vi "Begin.vi"(8 "error in":errorcluster) -> (0 "error out":errorcluster)   [LabVIEW 2017]
doc: "Called before other user functions, this VI is expected to open initial I/O refnums, load in file data, and do all program initialization. Notice that the <B>error out</B> terminal is simply used for data flow. Wiring it to other structures or subVIs ensures that this VI runs first."
uses:
  <vilib>/Rock Robotics/WPI/DriverStation/WPI_DriverStationRobotMode2.ctl
  TypeDef/CLUSTER_Arm_Device_IDs.ctl
  TypeDef/CLUSTER_Talon_Setup.ctl
  _SHARE ALL/RoboRio Share All/SRX Share All/TypeDefs SRX/Cluster_SRX_OPEN Data.ctl
  _SHARE ALL/RoboRio Share All/SRX Share All/TypeDefs SRX/Cluster_SRX_Current Config.ctl
  _SHARE ALL/RoboRio Share All/SRX Share All/TypeDefs SRX/Cluster_SRX_Sensor Config.ctl
  System Drivers/Phoenix-LabVIEW/Motor Controller/Controls/CTRE_Phoenix_MotorControl_FeedbackDevice.ctl
  _SHARE ALL/RoboRio Share All/SRX Share All/TypeDefs SRX/Cluster_SRX_Config Hard Limits.ctl
  System Drivers/Phoenix-LabVIEW/Motor Controller/Controls/CTRE_Phoenix_MotorControl_LimitSwitchNormal.ctl
  _SHARE ALL/RoboRio Share All/SRX Share All/TypeDefs SRX/Cluster_SRX_Motion Magic Config Data.ctl
  _SHARE ALL/RoboRio Share All/SRX Share All/TypeDefs SRX/Cluster_SRX_PIDF.ctl
  _SHARE ALL/RoboRio Share All/SRX Share All/TypeDefs SRX/Cluster_SRX_Config Soft Limits.ctl
  _SHARE ALL/RoboRio Share All/SRX Share All/TypeDefs SRX/Cluster_SRX_Config Voltage Output.ctl
  System Drivers/Phoenix-LabVIEW/Motor Controller/Controls/CTRE_Phoenix_MotorControl_NeutralMode.ctl
  _SHARE ALL/RoboRio Share All/SRX Share All/TypeDefs SRX/Cluster_SRX_Forward and Reverse.ctl
  TypeDef/CLUSTER_Claw_Setup.ctl
  TypeDef/CLUSTER_PWM Motor Setup.ctl
  TypeDef/CLUSTER_Solonoid_Setup.ctl
  <vilib>/Rock Robotics/WPI/Solenoid/WPI_SolenoidChannel.ctl
  <vilib>/Rock Robotics/SystemInterfaces/DIO/FPGA_DIOChannel.ctl
  TypeDef/CLUSTER_Drive_Setup.ctl
  Robot Global Data.vi
  _SHARE ALL/Global Share All/Global_STOP.vi
  Globals/Global_Device_IDs.vi
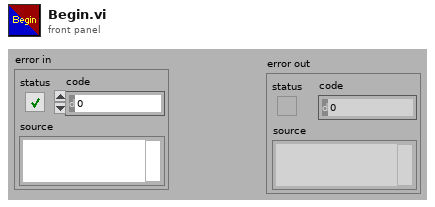
[diagram p1: front panel]
types:
  T1 = typedef "WPI_DriverStationRobotMode2.ctl" = enum16{"Autonomous Disabled", "Autonomous Enabled", "Teleop Disabled", "Teleop Enabled", "Disconnected", "Finish", "Test Disabled", "Test Enabled", "Emergency Stopped"}
  T2 = typedef "CTRE_Phoenix_MotorControl_LimitSwitchNormal.ctl" = enum16{"Normally Open", "Normally Closed", "Disabled"}
  T3 = typedef "Cluster_SRX_Config Hard Limits.ctl" = cluster{"Fwd Enable":bool, "Rev Enable":bool, "Fwd NO-NC":T2, "Rev NO-NC":T2}
  T4 = typedef "Cluster_SRX_Forward and Reverse.ctl" = cluster{"Forward":dbl, "Reverse":dbl}
  T5 = typedef "CTRE_Phoenix_MotorControl_NeutralMode.ctl" = enum8{"EEPROMSetting", "Override to Coast", "Override to Brake"}
  T6 = typedef "Cluster_SRX_Config Voltage Output.ctl" = cluster{"Invert?":bool, "Neutral Mode":T5, "Deadband (-1to1)":dbl, "Ramp Time Off to Full (S)":dbl, "Peak  (-1to1)":T4, "Nominal  (-1to1)":T4}
  T7 = typedef "Cluster_SRX_Config Soft Limits.ctl" = cluster{"Max":i32, "Min":i32, "Max Enable":bool, "Min Enable":bool}
  T8 = typedef "Cluster_SRX_PIDF.ctl" = cluster{"P":dbl, "I":dbl, "D":dbl, "F":dbl, "I Zone":dbl}
  T9 = typedef "Cluster_SRX_Sensor Config.ctl" = cluster{"Feedback Device":T10, "PhaseSensor":bool}
  T10 = typedef "CTRE_Phoenix_MotorControl_FeedbackDevice.ctl" = i8
  T11 = typedef "Cluster_SRX_OPEN Data.ctl" = cluster{"SRX ID":u8, "Invert Output":bool}
  T12 = typedef "CLUSTER_Talon_Setup.ctl" = cluster{"Open Data":T11, "Current Config Data":T13, "Sensor Config":T9, "Hard Limits":T3, "Motion Magic Config Data":T14, "PIDF":T8, "Maximum Integral Accumulator Value":dbl, "AllowableClosedLoop":i32, "Limits":T7, "Output Config":T6}
  T13 = typedef "Cluster_SRX_Current Config.ctl" = cluster{"Enable Current Limit?":bool, "Peak Current (Amps)":i32, "Peak Current Maximum Duration (ms)":i32, "Continuous Current Limit (Amps)":i32}
  T14 = typedef "Cluster_SRX_Motion Magic Config Data.ctl" = cluster{"Cruise Velocity":i32, "Acceleration":i32}
  T15 = typedef "CLUSTER_Arm_Device_IDs.ctl" = cluster{"Master":T12, "Slave":T12}
  T16 = typedef "CLUSTER_Drive_Setup.ctl" = cluster{"Left Master":T12, "Right Master":T12, "Left Slave":T12, "Right Slave":T12}
  T17 = typedef "FPGA_DIOChannel.ctl" = enum8{"DIO 0", "DIO 1", "DIO 2", "DIO 3", "DIO 4", "DIO 5", "DIO 6", "DIO 7", "DIO 8", "DIO 9", "DIO MXP 0", "DIO MXP 1", "DIO MXP 2", "DIO MXP 3", "DIO MXP 4", "DIO MXP 5", "DIO MXP 6", "DIO MXP 7", "DIO MXP 8", "DIO MXP 9", "DIO MXP 10", "DIO MXP 11", "DIO MXP 12", "DIO MXP 13", "DIO MXP 14", "DIO MXP 15", "SPI Port CS1", "SPI Port CS2", "SPI Port CS3", "SPI Port MISO", "SPI Port MOSI", "Invalid"}
  T18 = typedef "WPI_SolenoidChannel.ctl" = enum8{"Solenoid 0", "Solenoid 1", "Solenoid 2", "Solenoid 3", "Solenoid 4", "Solenoid 5", "Solenoid 6", "Solenoid 7", "Invalid"}
  T19 = typedef "CLUSTER_Claw_Setup.ctl" = cluster{"Left Motor Setup":T20, "Right Motor Setup":T20, "Left Motor PDP":i32, "Right Motor PDP":i32, "Solonoid Setup":T21, "Limit Switch DIO":T17}
  T20 = typedef "CLUSTER_PWM Motor Setup.ctl" = cluster{"Motor ID":u8, "Invert Motor":bool}
  T21 = typedef "CLUSTER_Solonoid_Setup.ctl" = cluster{"Pneumatics Control Module (0)":u8, "Forward Solenoid Channel":T18, "Reverse Solenoid Channel":T18}
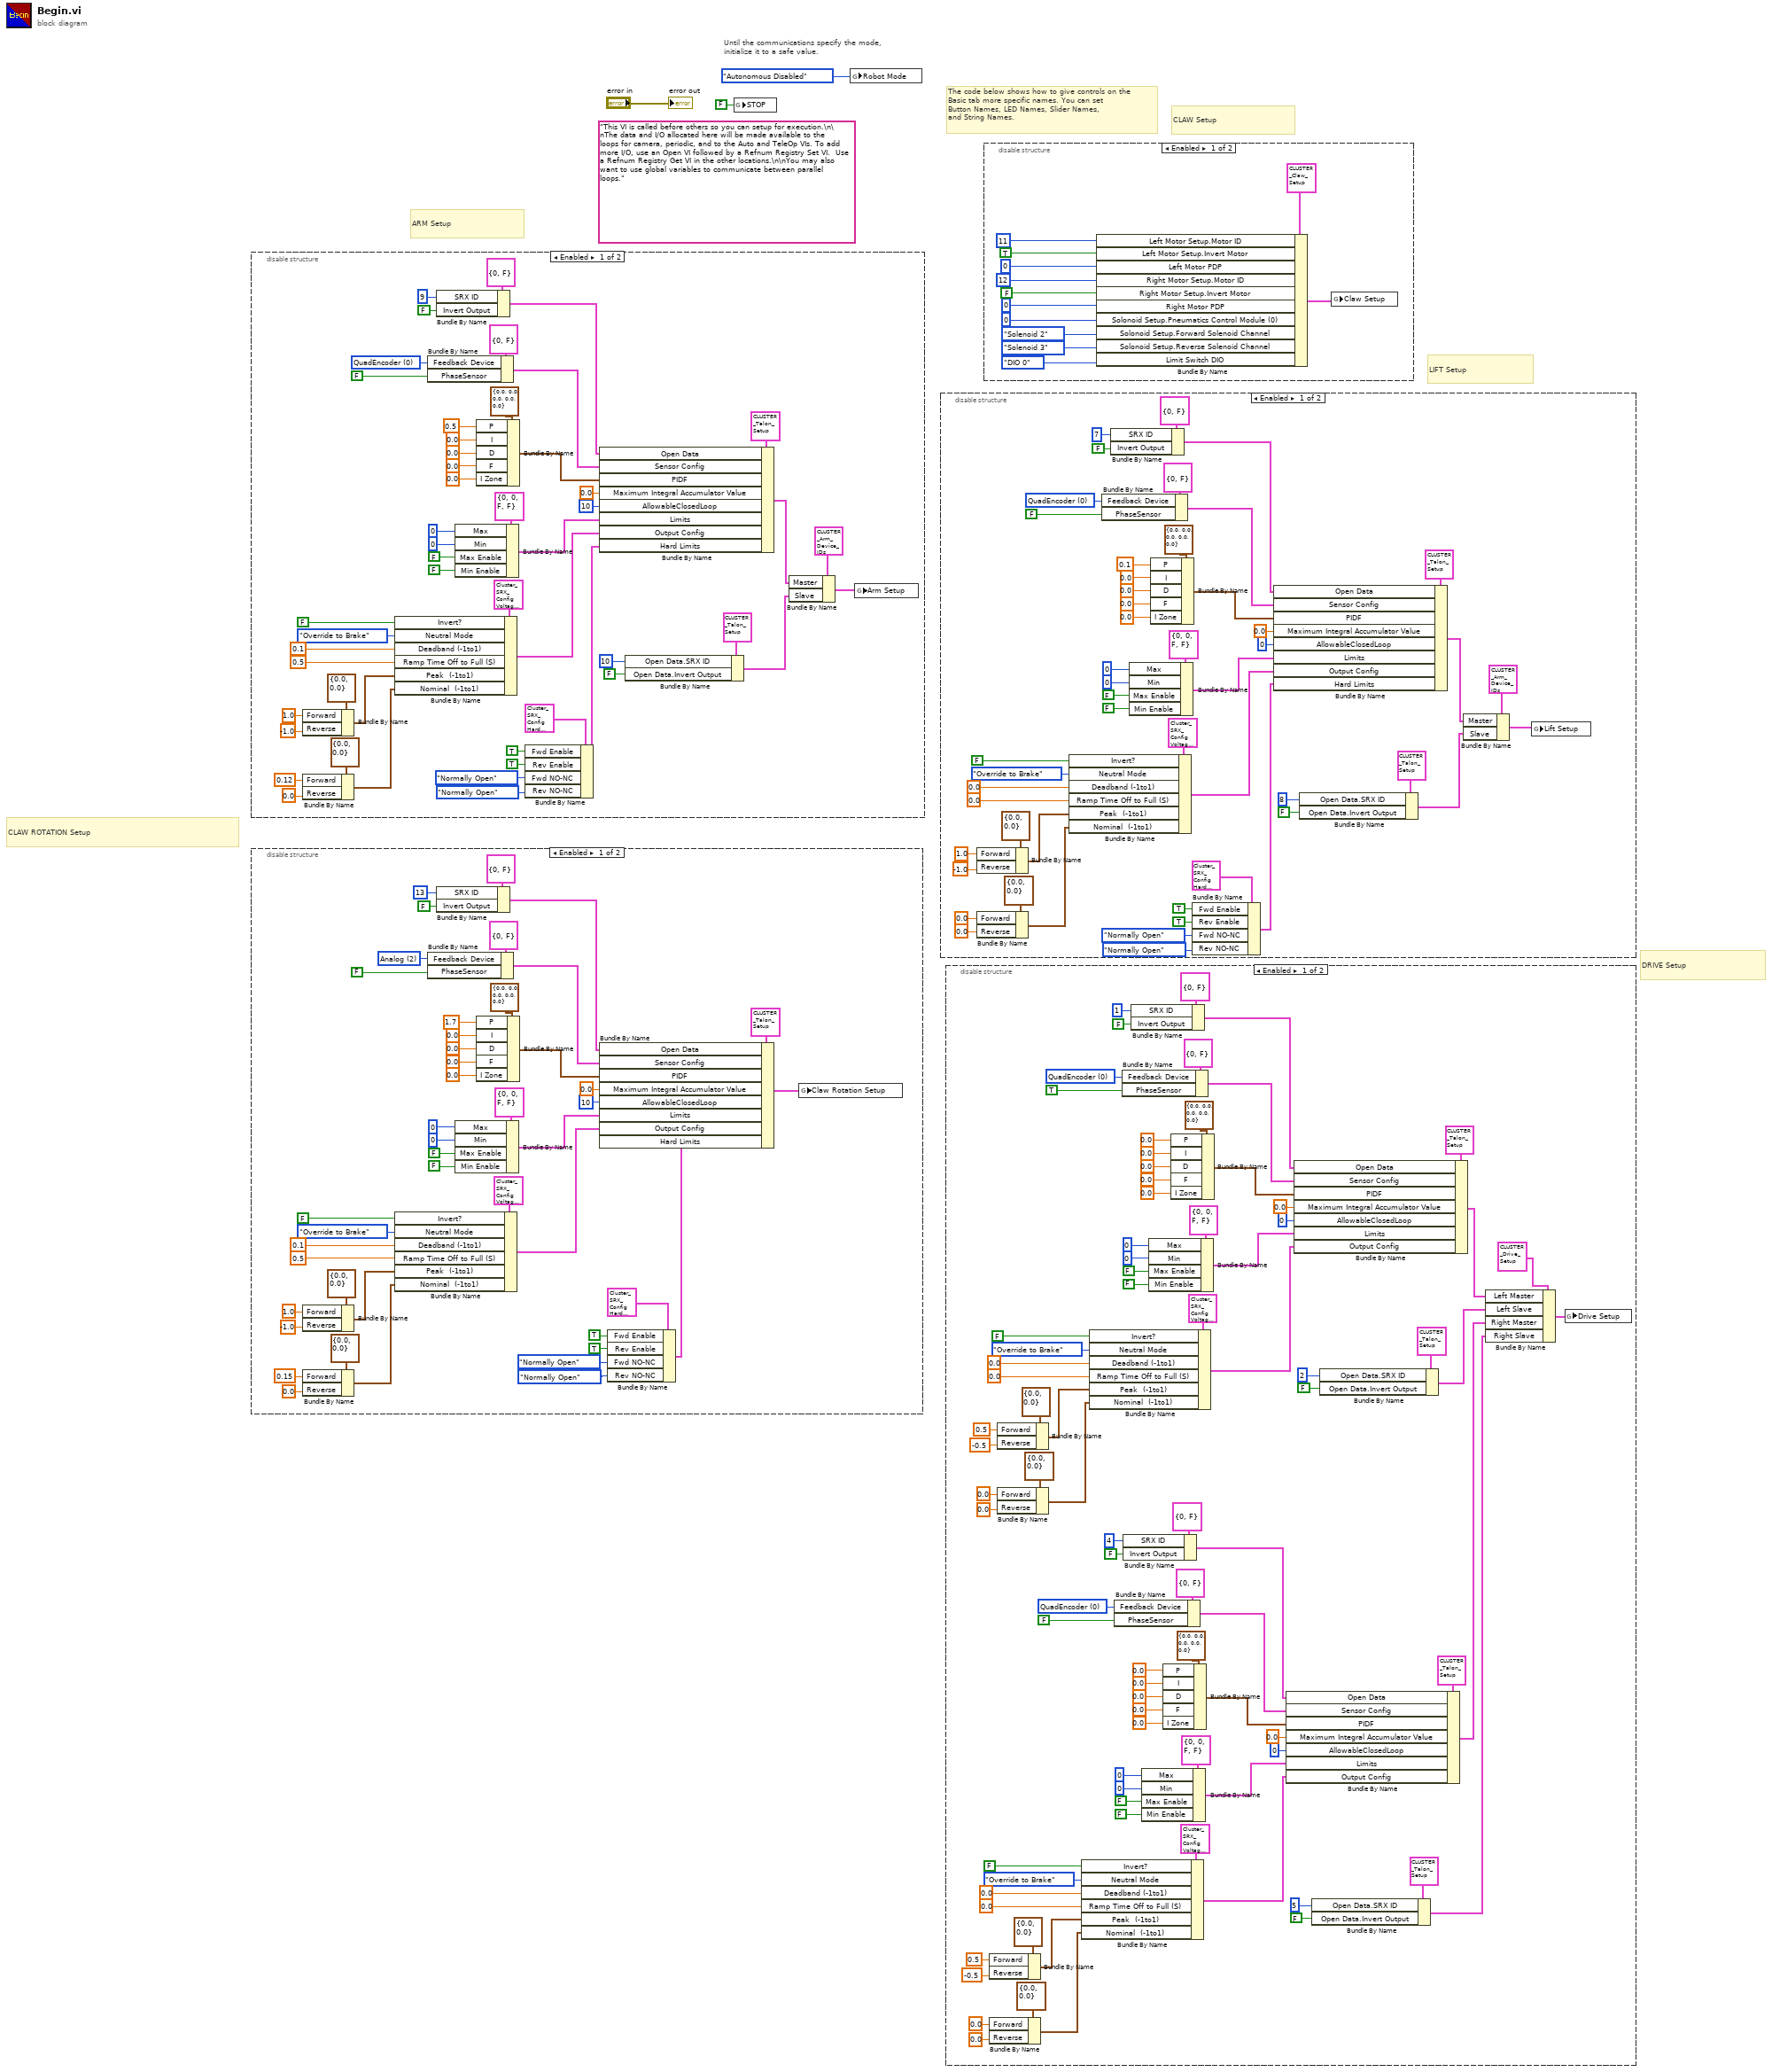
[diagram p0: block diagram]
diagram:
  (unwired) "This VI is called before others so you can setup for execution.\n\nThe data and I/O allocated here will be made available to the loops for camera, periodic, and to the Auto and TeleOp VIs. To add more I/O, use an Open VI followed by a Refnum Registry Set VI.  Use a Refnum Registry Get VI in the other locations.\n\nYou may also want to use global variables to communicate between parallel loops."
  # "DRIVE Setup"
  # "CLAW ROTATION Setup"
  # "LIFT Setup"
  # "CLAW Setup"
  # "ARM Setup"
  # "The code below shows how to give controls on the\nBasic tab more specific names. You can set\nButton Names, LED Names, Slider Names,\nand String Names."
  # "Until the communications specify the mode,\ninitialize it to a safe value."
  n1 = disable-structure shown="Enabled" {
    frame Enabled {
      w34 = T10 0 items=["None"=-1, "QuadEncoder"=0, "Analog"=2, "Tachometer"=4, "Pulse Width Encoded Position"=8, "Sensor Sum (S0 + S1)"=9, "Sensor Difference (D0 - D1)"=10, "Remote Source 0"=11, "Remote Source 1"=12, "Software Emulated"=15] ("Feedback Device")
      n2 = Bundle By Name(cluster=T4 {"Forward"=0.0, "Reverse"=0.0} ("Peak  (-1to1)"), "Forward"=1.0, "Reverse"=-1.0) -> (w18:T4)
      n3 = Bundle By Name(cluster=T4 {"Forward"=0.0, "Reverse"=0.0} ("Nominal  (-1to1)"), "Forward"=0.12, "Reverse"=0.0) -> (w16:T4)
      n4 = Bundle By Name(cluster=T6 {"Invert?"=FALSE, "Neutral Mode"=enum."Override to Coast", "Deadband (-1to1)"=0.0, "Ramp Time Off to Full (S)"=0.0, "Peak  (-1to1)"={"Forward"=1.0, "Reverse"=-1.0}, "Nominal  (-1to1)"={"Forward"=0.0, "Reverse"=0.0}} ("Output Config"), "Invert?"=FALSE, "Neutral Mode"=CTRE_Phoenix_MotorControl_NeutralMode."Override to Brake", "Deadband (-1to1)"=0.1, "Ramp Time Off to Full (S)"=0.5, "Peak  (-1to1)"=w18, "Nominal  (-1to1)"=w16) -> (w37:T6)
      n5 = Bundle By Name(cluster=T9 {"Feedback Device"=0, "PhaseSensor"=FALSE} ("Sensor Config"), "Feedback Device"=w34, "PhaseSensor"=FALSE) -> (w45:T9)
      n6 = Bundle By Name(cluster=T11 {"SRX ID"=0, "Invert Output"=FALSE} ("Open Data"), "SRX ID"=u8 9, "Invert Output"=FALSE) -> (w47:T11)
      n7 = Bundle By Name(cluster=T7 {"Max"=0, "Min"=0, "Max Enable"=FALSE, "Min Enable"=FALSE} ("Limits"), "Max"=0, "Min"=0, "Max Enable"=FALSE, "Min Enable"=FALSE) -> (w39:T7)
      n8 = Bundle By Name(cluster=T8 {"P"=0.0, "I"=0.0, "D"=0.0, "F"=0.0, "I Zone"=0.0} ("PIDF"), "P"=0.5, "I"=0.0, "D"=0.0, "F"=0.0, "I Zone"=0.0) -> (w43:T8)
      n9 = Bundle By Name(cluster=T3 {"Fwd Enable"=FALSE, "Rev Enable"=FALSE, "Fwd NO-NC"=enum."Normally Open", "Rev NO-NC"=enum."Normally Open"} ("Hard Limits"), "Fwd Enable"=TRUE, "Rev Enable"=TRUE, "Fwd NO-NC"=CTRE_Phoenix_MotorControl_LimitSwitchNormal."Normally Open", "Rev NO-NC"=CTRE_Phoenix_MotorControl_LimitSwitchNormal."Normally Open") -> (w4:T3)
      n10 = Bundle By Name(cluster=T12 {"Open Data"={"SRX ID"=0, "Invert Output"=FALSE}, "Current Config Data"={"Enable Current Limit?"=FALSE, "Peak Current (Amps)"=0, "Peak Current Maximum Duration (ms)"=0, "Continuous Current Limit (Amps)"=0}, "Sensor Config"={"Feedback Device"=0, "PhaseSensor"=FALSE}, "Hard Limits"={"Fwd Enable"=FALSE, "Rev Enable"=FALSE, "Fwd NO-NC"=enum."Normally Open", "Rev NO-NC"=enum."Normally Open"}, "Motion Magic Config Data"={"Cruise Velocity"=0, "Acceleration"=0}, "PIDF"={"P"=0.0, "I"=0.0, "D"=0.0, "F"=0.0, "I Zone"=0.0}, "Maximum Integral Accumulator Value"=0.0, "AllowableClosedLoop"=0, "Limits"={"Max"=0, "Min"=0, "Max Enable"=FALSE, "Min Enable"=FALSE}, "Output Config"={"Invert?"=FALSE, "Neutral Mode"=enum."Override to Coast", "Deadband (-1to1)"=0.0, "Ramp Time Off to Full (S)"=0.0, "Peak  (-1to1)"={"Forward"=1.0, "Reverse"=-1.0}, "Nominal  (-1to1)"={"Forward"=0.0, "Reverse"=0.0}}} ("Master"), "Open Data"=w47, "Sensor Config"=w45, "PIDF"=w43, "Maximum Integral Accumulator Value"=0.0, "AllowableClosedLoop"=10, "Limits"=w39, "Output Config"=w37, "Hard Limits"=w4) -> (w51:T12)
      n11 = Bundle By Name(cluster=T12 {"Open Data"={"SRX ID"=0, "Invert Output"=FALSE}, "Current Config Data"={"Enable Current Limit?"=FALSE, "Peak Current (Amps)"=0, "Peak Current Maximum Duration (ms)"=0, "Continuous Current Limit (Amps)"=0}, "Sensor Config"={"Feedback Device"=0, "PhaseSensor"=FALSE}, "Hard Limits"={"Fwd Enable"=FALSE, "Rev Enable"=FALSE, "Fwd NO-NC"=enum."Normally Open", "Rev NO-NC"=enum."Normally Open"}, "Motion Magic Config Data"={"Cruise Velocity"=0, "Acceleration"=0}, "PIDF"={"P"=0.0, "I"=0.0, "D"=0.0, "F"=0.0, "I Zone"=0.0}, "Maximum Integral Accumulator Value"=0.0, "AllowableClosedLoop"=0, "Limits"={"Max"=0, "Min"=0, "Max Enable"=FALSE, "Min Enable"=FALSE}, "Output Config"={"Invert?"=FALSE, "Neutral Mode"=enum."Override to Coast", "Deadband (-1to1)"=0.0, "Ramp Time Off to Full (S)"=0.0, "Peak  (-1to1)"={"Forward"=1.0, "Reverse"=-1.0}, "Nominal  (-1to1)"={"Forward"=0.0, "Reverse"=0.0}}} ("Master"), "Open Data.SRX ID"=u8 10, "Open Data.Invert Output"=FALSE) -> (w50:T12)
      n12 = Bundle By Name(cluster=T15 {"Master"={"Open Data"={"SRX ID"=0, "Invert Output"=FALSE}, "Current Config Data"={"Enable Current Limit?"=FALSE, "Peak Current (Amps)"=0, "Peak Current Maximum Duration (ms)"=2, "Continuous Current Limit (Amps)"=0}, "Sensor Config"={"Feedback Device"=0, "PhaseSensor"=FALSE}, "Hard Limits"={"Fwd Enable"=FALSE, "Rev Enable"=FALSE, "Fwd NO-NC"=enum."Normally Open", "Rev NO-NC"=enum."Normally Open"}, "Motion Magic Config Data"={"Cruise Velocity"=0, "Acceleration"=0}, "PIDF"={"P"=0.0, "I"=0.0, "D"=0.0, "F"=0.0, "I Zone"=0.0}, "Maximum Integral Accumulator Value"=0.0, "AllowableClosedLoop"=0, "Limits"={"Max"=0, "Min"=0, "Max Enable"=FALSE, "Min Enable"=FALSE}, "Output Config"={"Invert?"=FALSE, "Neutral Mode"=enum."Override to Coast", "Deadband (-1to1)"=0.0, "Ramp Time Off to Full (S)"=0.0, "Peak  (-1to1)"={"Forward"=1.0, "Reverse"=-1.0}, "Nominal  (-1to1)"={"Forward"=0.0, "Reverse"=0.0}}}, "Slave"={"Open Data"={"SRX ID"=0, "Invert Output"=FALSE}, "Current Config Data"={"Enable Current Limit?"=FALSE, "Peak Current (Amps)"=0, "Peak Current Maximum Duration (ms)"=-1, "Continuous Current Limit (Amps)"=0}, "Sensor Config"={"Feedback Device"=0, "PhaseSensor"=FALSE}, "Hard Limits"={"Fwd Enable"=FALSE, "Rev Enable"=FALSE, "Fwd NO-NC"=enum."Normally Open", "Rev NO-NC"=enum."Normally Open"}, "Motion Magic Config Data"={"Cruise Velocity"=0, "Acceleration"=0}, "PIDF"={"P"=0.0, "I"=0.0, "D"=0.0, "F"=0.0, "I Zone"=0.0}, "Maximum Integral Accumulator Value"=0.0, "AllowableClosedLoop"=0, "Limits"={"Max"=0, "Min"=0, "Max Enable"=FALSE, "Min Enable"=FALSE}, "Output Config"={"Invert?"=FALSE, "Neutral Mode"=enum."Override to Coast", "Deadband (-1to1)"=0.0, "Ramp Time Off to Full (S)"=0.0, "Peak  (-1to1)"={"Forward"=1.0, "Reverse"=-1.0}, "Nominal  (-1to1)"={"Forward"=0.0, "Reverse"=0.0}}}} ("Arm Setup"), "Master"=w51, "Slave"=w50) -> (w53:T15)
      n13 = global write "Global_Device_IDs.vi" "Arm Setup"(w53) -> ()
    }
    frame Disabled {
    }
  }
  n14 = disable-structure shown="Enabled" {
    frame Enabled {
      w84 = T10 2 items=["None"=-1, "QuadEncoder"=0, "Analog"=2, "Tachometer"=4, "Pulse Width Encoded Position"=8, "Sensor Sum (S0 + S1)"=9, "Sensor Difference (D0 - D1)"=10, "Remote Source 0"=11, "Remote Source 1"=12, "Software Emulated"=15] ("Feedback Device")
      n15 = Bundle By Name(cluster=T4 {"Forward"=0.0, "Reverse"=0.0} ("Peak  (-1to1)"), "Forward"=1.0, "Reverse"=-1.0) -> (w68:T4)
      n16 = Bundle By Name(cluster=T4 {"Forward"=0.0, "Reverse"=0.0} ("Nominal  (-1to1)"), "Forward"=0.15, "Reverse"=0.0) -> (w66:T4)
      n17 = Bundle By Name(cluster=T6 {"Invert?"=FALSE, "Neutral Mode"=enum."Override to Coast", "Deadband (-1to1)"=0.0, "Ramp Time Off to Full (S)"=0.0, "Peak  (-1to1)"={"Forward"=1.0, "Reverse"=-1.0}, "Nominal  (-1to1)"={"Forward"=0.0, "Reverse"=0.0}} ("Output Config"), "Invert?"=FALSE, "Neutral Mode"=CTRE_Phoenix_MotorControl_NeutralMode."Override to Brake", "Deadband (-1to1)"=0.1, "Ramp Time Off to Full (S)"=0.5, "Peak  (-1to1)"=w68, "Nominal  (-1to1)"=w66) -> (w87:T6)
      n18 = Bundle By Name(cluster=T9 {"Feedback Device"=0, "PhaseSensor"=FALSE} ("Sensor Config"), "Feedback Device"=w84, "PhaseSensor"=FALSE) -> (w95:T9)
      n19 = Bundle By Name(cluster=T11 {"SRX ID"=0, "Invert Output"=FALSE} ("Open Data"), "SRX ID"=u8 13, "Invert Output"=FALSE) -> (w97:T11)
      n20 = Bundle By Name(cluster=T7 {"Max"=0, "Min"=0, "Max Enable"=FALSE, "Min Enable"=FALSE} ("Limits"), "Max"=0, "Min"=0, "Max Enable"=FALSE, "Min Enable"=FALSE) -> (w89:T7)
      n21 = Bundle By Name(cluster=T8 {"P"=0.0, "I"=0.0, "D"=0.0, "F"=0.0, "I Zone"=0.0} ("PIDF"), "P"=1.7, "I"=0.0, "D"=0.0, "F"=0.0, "I Zone"=0.0) -> (w93:T8)
      n22 = Bundle By Name(cluster=T3 {"Fwd Enable"=FALSE, "Rev Enable"=FALSE, "Fwd NO-NC"=enum."Normally Open", "Rev NO-NC"=enum."Normally Open"} ("Hard Limits"), "Fwd Enable"=TRUE, "Rev Enable"=TRUE, "Fwd NO-NC"=CTRE_Phoenix_MotorControl_LimitSwitchNormal."Normally Open", "Rev NO-NC"=CTRE_Phoenix_MotorControl_LimitSwitchNormal."Normally Open") -> (w56:T3)
      n23 = Bundle By Name(cluster=T12 {"Open Data"={"SRX ID"=0, "Invert Output"=FALSE}, "Current Config Data"={"Enable Current Limit?"=FALSE, "Peak Current (Amps)"=0, "Peak Current Maximum Duration (ms)"=0, "Continuous Current Limit (Amps)"=0}, "Sensor Config"={"Feedback Device"=0, "PhaseSensor"=FALSE}, "Hard Limits"={"Fwd Enable"=FALSE, "Rev Enable"=FALSE, "Fwd NO-NC"=enum."Normally Open", "Rev NO-NC"=enum."Normally Open"}, "Motion Magic Config Data"={"Cruise Velocity"=0, "Acceleration"=0}, "PIDF"={"P"=0.0, "I"=0.0, "D"=0.0, "F"=0.0, "I Zone"=0.0}, "Maximum Integral Accumulator Value"=0.0, "AllowableClosedLoop"=0, "Limits"={"Max"=0, "Min"=0, "Max Enable"=FALSE, "Min Enable"=FALSE}, "Output Config"={"Invert?"=FALSE, "Neutral Mode"=enum."Override to Coast", "Deadband (-1to1)"=0.0, "Ramp Time Off to Full (S)"=0.0, "Peak  (-1to1)"={"Forward"=1.0, "Reverse"=-1.0}, "Nominal  (-1to1)"={"Forward"=0.0, "Reverse"=0.0}}} ("Master"), "Open Data"=w97, "Sensor Config"=w95, "PIDF"=w93, "Maximum Integral Accumulator Value"=0.0, "AllowableClosedLoop"=10, "Limits"=w89, "Output Config"=w87, "Hard Limits"=w56) -> (w61:T12)
      n24 = global write "Global_Device_IDs.vi" "Claw Rotation Setup"(w61) -> ()
    }
    frame Disabled {
    }
  }
  n25 = global write "Global_STOP.vi" "STOP"(FALSE ("STOP")) -> ()
  n26 = global write "Robot Global Data.vi" "Robot Mode"(WPI_DriverStationRobotMode2."Autonomous Disabled" ("Robot Mode")) -> ()
  n27 = disable-structure shown="Enabled" {
    frame Enabled {
      w130 = T10 0 items=["None"=-1, "QuadEncoder"=0, "Analog"=2, "Tachometer"=4, "Pulse Width Encoded Position"=8, "Sensor Sum (S0 + S1)"=9, "Sensor Difference (D0 - D1)"=10, "Remote Source 0"=11, "Remote Source 1"=12, "Software Emulated"=15] ("Feedback Device")
      n28 = Bundle By Name(cluster=T4 {"Forward"=0.0, "Reverse"=0.0} ("Peak  (-1to1)"), "Forward"=1.0, "Reverse"=-1.0) -> (w114:T4)
      n29 = Bundle By Name(cluster=T4 {"Forward"=0.0, "Reverse"=0.0} ("Nominal  (-1to1)"), "Forward"=0.0, "Reverse"=0.0) -> (w112:T4)
      n30 = Bundle By Name(cluster=T6 {"Invert?"=FALSE, "Neutral Mode"=enum."Override to Coast", "Deadband (-1to1)"=0.0, "Ramp Time Off to Full (S)"=0.0, "Peak  (-1to1)"={"Forward"=1.0, "Reverse"=-1.0}, "Nominal  (-1to1)"={"Forward"=0.0, "Reverse"=0.0}} ("Output Config"), "Invert?"=FALSE, "Neutral Mode"=CTRE_Phoenix_MotorControl_NeutralMode."Override to Brake", "Deadband (-1to1)"=0.0, "Ramp Time Off to Full (S)"=0.0, "Peak  (-1to1)"=w114, "Nominal  (-1to1)"=w112) -> (w133:T6)
      n31 = Bundle By Name(cluster=T9 {"Feedback Device"=0, "PhaseSensor"=FALSE} ("Sensor Config"), "Feedback Device"=w130, "PhaseSensor"=FALSE) -> (w141:T9)
      n32 = Bundle By Name(cluster=T11 {"SRX ID"=0, "Invert Output"=FALSE} ("Open Data"), "SRX ID"=u8 7, "Invert Output"=FALSE) -> (w143:T11)
      n33 = Bundle By Name(cluster=T7 {"Max"=0, "Min"=0, "Max Enable"=FALSE, "Min Enable"=FALSE} ("Limits"), "Max"=0, "Min"=0, "Max Enable"=FALSE, "Min Enable"=FALSE) -> (w135:T7)
      n34 = Bundle By Name(cluster=T8 {"P"=0.0, "I"=0.0, "D"=0.0, "F"=0.0, "I Zone"=0.0} ("PIDF"), "P"=0.1, "I"=0.0, "D"=0.0, "F"=0.0, "I Zone"=0.0) -> (w139:T8)
      n35 = Bundle By Name(cluster=T3 {"Fwd Enable"=FALSE, "Rev Enable"=FALSE, "Fwd NO-NC"=enum."Normally Open", "Rev NO-NC"=enum."Normally Open"} ("Hard Limits"), "Fwd Enable"=TRUE, "Rev Enable"=TRUE, "Fwd NO-NC"=CTRE_Phoenix_MotorControl_LimitSwitchNormal."Normally Open", "Rev NO-NC"=CTRE_Phoenix_MotorControl_LimitSwitchNormal."Normally Open") -> (w105:T3)
      n36 = Bundle By Name(cluster=T12 {"Open Data"={"SRX ID"=0, "Invert Output"=FALSE}, "Current Config Data"={"Enable Current Limit?"=FALSE, "Peak Current (Amps)"=0, "Peak Current Maximum Duration (ms)"=0, "Continuous Current Limit (Amps)"=0}, "Sensor Config"={"Feedback Device"=0, "PhaseSensor"=FALSE}, "Hard Limits"={"Fwd Enable"=FALSE, "Rev Enable"=FALSE, "Fwd NO-NC"=enum."Normally Open", "Rev NO-NC"=enum."Normally Open"}, "Motion Magic Config Data"={"Cruise Velocity"=0, "Acceleration"=0}, "PIDF"={"P"=0.0, "I"=0.0, "D"=0.0, "F"=0.0, "I Zone"=0.0}, "Maximum Integral Accumulator Value"=0.0, "AllowableClosedLoop"=0, "Limits"={"Max"=0, "Min"=0, "Max Enable"=FALSE, "Min Enable"=FALSE}, "Output Config"={"Invert?"=FALSE, "Neutral Mode"=enum."Override to Coast", "Deadband (-1to1)"=0.0, "Ramp Time Off to Full (S)"=0.0, "Peak  (-1to1)"={"Forward"=1.0, "Reverse"=-1.0}, "Nominal  (-1to1)"={"Forward"=0.0, "Reverse"=0.0}}} ("Master"), "Open Data"=w143, "Sensor Config"=w141, "PIDF"=w139, "Maximum Integral Accumulator Value"=0.0, "AllowableClosedLoop"=0, "Limits"=w135, "Output Config"=w133, "Hard Limits"=w105) -> (w147:T12)
      n37 = Bundle By Name(cluster=T12 {"Open Data"={"SRX ID"=0, "Invert Output"=FALSE}, "Current Config Data"={"Enable Current Limit?"=FALSE, "Peak Current (Amps)"=0, "Peak Current Maximum Duration (ms)"=0, "Continuous Current Limit (Amps)"=0}, "Sensor Config"={"Feedback Device"=0, "PhaseSensor"=FALSE}, "Hard Limits"={"Fwd Enable"=FALSE, "Rev Enable"=FALSE, "Fwd NO-NC"=enum."Normally Open", "Rev NO-NC"=enum."Normally Open"}, "Motion Magic Config Data"={"Cruise Velocity"=0, "Acceleration"=0}, "PIDF"={"P"=0.0, "I"=0.0, "D"=0.0, "F"=0.0, "I Zone"=0.0}, "Maximum Integral Accumulator Value"=0.0, "AllowableClosedLoop"=0, "Limits"={"Max"=0, "Min"=0, "Max Enable"=FALSE, "Min Enable"=FALSE}, "Output Config"={"Invert?"=FALSE, "Neutral Mode"=enum."Override to Coast", "Deadband (-1to1)"=0.0, "Ramp Time Off to Full (S)"=0.0, "Peak  (-1to1)"={"Forward"=1.0, "Reverse"=-1.0}, "Nominal  (-1to1)"={"Forward"=0.0, "Reverse"=0.0}}} ("Master"), "Open Data.SRX ID"=u8 8, "Open Data.Invert Output"=FALSE) -> (w146:T12)
      n38 = Bundle By Name(cluster=T15 {"Master"={"Open Data"={"SRX ID"=0, "Invert Output"=FALSE}, "Current Config Data"={"Enable Current Limit?"=FALSE, "Peak Current (Amps)"=0, "Peak Current Maximum Duration (ms)"=2, "Continuous Current Limit (Amps)"=0}, "Sensor Config"={"Feedback Device"=0, "PhaseSensor"=FALSE}, "Hard Limits"={"Fwd Enable"=FALSE, "Rev Enable"=FALSE, "Fwd NO-NC"=enum."Normally Open", "Rev NO-NC"=enum."Normally Open"}, "Motion Magic Config Data"={"Cruise Velocity"=0, "Acceleration"=0}, "PIDF"={"P"=0.0, "I"=0.0, "D"=0.0, "F"=0.0, "I Zone"=0.0}, "Maximum Integral Accumulator Value"=0.0, "AllowableClosedLoop"=0, "Limits"={"Max"=0, "Min"=0, "Max Enable"=FALSE, "Min Enable"=FALSE}, "Output Config"={"Invert?"=FALSE, "Neutral Mode"=enum."Override to Coast", "Deadband (-1to1)"=0.0, "Ramp Time Off to Full (S)"=0.0, "Peak  (-1to1)"={"Forward"=1.0, "Reverse"=-1.0}, "Nominal  (-1to1)"={"Forward"=0.0, "Reverse"=0.0}}}, "Slave"={"Open Data"={"SRX ID"=0, "Invert Output"=FALSE}, "Current Config Data"={"Enable Current Limit?"=FALSE, "Peak Current (Amps)"=0, "Peak Current Maximum Duration (ms)"=-1, "Continuous Current Limit (Amps)"=0}, "Sensor Config"={"Feedback Device"=0, "PhaseSensor"=FALSE}, "Hard Limits"={"Fwd Enable"=FALSE, "Rev Enable"=FALSE, "Fwd NO-NC"=enum."Normally Open", "Rev NO-NC"=enum."Normally Open"}, "Motion Magic Config Data"={"Cruise Velocity"=0, "Acceleration"=0}, "PIDF"={"P"=0.0, "I"=0.0, "D"=0.0, "F"=0.0, "I Zone"=0.0}, "Maximum Integral Accumulator Value"=0.0, "AllowableClosedLoop"=0, "Limits"={"Max"=0, "Min"=0, "Max Enable"=FALSE, "Min Enable"=FALSE}, "Output Config"={"Invert?"=FALSE, "Neutral Mode"=enum."Override to Coast", "Deadband (-1to1)"=0.0, "Ramp Time Off to Full (S)"=0.0, "Peak  (-1to1)"={"Forward"=1.0, "Reverse"=-1.0}, "Nominal  (-1to1)"={"Forward"=0.0, "Reverse"=0.0}}}} ("Arm Setup"), "Master"=w147, "Slave"=w146) -> (w149:T15)
      n39 = global write "Global_Device_IDs.vi" "Lift Setup"(w149) -> ()
    }
    frame Disabled {
    }
  }
  n40 = disable-structure shown="Enabled" {
    frame Enabled {
      w170 = T10 0 items=["None"=-1, "QuadEncoder"=0, "Analog"=2, "Tachometer"=4, "Pulse Width Encoded Position"=8, "Sensor Sum (S0 + S1)"=9, "Sensor Difference (D0 - D1)"=10, "Remote Source 0"=11, "Remote Source 1"=12, "Software Emulated"=15] ("Feedback Device")
      w220 = T10 0 items=["None"=-1, "QuadEncoder"=0, "Analog"=2, "Tachometer"=4, "Pulse Width Encoded Position"=8, "Sensor Sum (S0 + S1)"=9, "Sensor Difference (D0 - D1)"=10, "Remote Source 0"=11, "Remote Source 1"=12, "Software Emulated"=15] ("Feedback Device")
      n41 = Bundle By Name(cluster=T4 {"Forward"=0.0, "Reverse"=0.0} ("Peak  (-1to1)"), "Forward"=0.5, "Reverse"=-0.5) -> (w186:T4)
      n42 = Bundle By Name(cluster=T4 {"Forward"=0.0, "Reverse"=0.0} ("Nominal  (-1to1)"), "Forward"=0.0, "Reverse"=0.0) -> (w188:T4)
      n43 = Bundle By Name(cluster=T4 {"Forward"=0.0, "Reverse"=0.0} ("Peak  (-1to1)"), "Forward"=0.5, "Reverse"=-0.5) -> (w204:T4)
      n44 = Bundle By Name(cluster=T4 {"Forward"=0.0, "Reverse"=0.0} ("Nominal  (-1to1)"), "Forward"=0.0, "Reverse"=0.0) -> (w202:T4)
      n45 = Bundle By Name(cluster=T6 {"Invert?"=FALSE, "Neutral Mode"=enum."Override to Coast", "Deadband (-1to1)"=0.0, "Ramp Time Off to Full (S)"=0.0, "Peak  (-1to1)"={"Forward"=1.0, "Reverse"=-1.0}, "Nominal  (-1to1)"={"Forward"=0.0, "Reverse"=0.0}} ("Output Config"), "Invert?"=FALSE, "Neutral Mode"=CTRE_Phoenix_MotorControl_NeutralMode."Override to Brake", "Deadband (-1to1)"=0.0, "Ramp Time Off to Full (S)"=0.0, "Peak  (-1to1)"=w186, "Nominal  (-1to1)"=w188) -> (w167:T6)
      n46 = Bundle By Name(cluster=T6 {"Invert?"=FALSE, "Neutral Mode"=enum."Override to Coast", "Deadband (-1to1)"=0.0, "Ramp Time Off to Full (S)"=0.0, "Peak  (-1to1)"={"Forward"=1.0, "Reverse"=-1.0}, "Nominal  (-1to1)"={"Forward"=0.0, "Reverse"=0.0}} ("Output Config"), "Invert?"=FALSE, "Neutral Mode"=CTRE_Phoenix_MotorControl_NeutralMode."Override to Brake", "Deadband (-1to1)"=0.0, "Ramp Time Off to Full (S)"=0.0, "Peak  (-1to1)"=w204, "Nominal  (-1to1)"=w202) -> (w223:T6)
      n47 = Bundle By Name(cluster=T9 {"Feedback Device"=0, "PhaseSensor"=FALSE} ("Sensor Config"), "Feedback Device"=w170, "PhaseSensor"=FALSE) -> (w159:T9)
      n48 = Bundle By Name(cluster=T9 {"Feedback Device"=0, "PhaseSensor"=FALSE} ("Sensor Config"), "Feedback Device"=w220, "PhaseSensor"=TRUE) -> (w231:T9)
      n49 = Bundle By Name(cluster=T11 {"SRX ID"=0, "Invert Output"=FALSE} ("Open Data"), "SRX ID"=u8 4, "Invert Output"=FALSE) -> (w157:T11)
      n50 = Bundle By Name(cluster=T11 {"SRX ID"=0, "Invert Output"=FALSE} ("Open Data"), "SRX ID"=u8 1, "Invert Output"=FALSE) -> (w233:T11)
      n51 = Bundle By Name(cluster=T7 {"Max"=0, "Min"=0, "Max Enable"=FALSE, "Min Enable"=FALSE} ("Limits"), "Max"=0, "Min"=0, "Max Enable"=FALSE, "Min Enable"=FALSE) -> (w165:T7)
      n52 = Bundle By Name(cluster=T7 {"Max"=0, "Min"=0, "Max Enable"=FALSE, "Min Enable"=FALSE} ("Limits"), "Max"=0, "Min"=0, "Max Enable"=FALSE, "Min Enable"=FALSE) -> (w225:T7)
      n53 = Bundle By Name(cluster=T8 {"P"=0.0, "I"=0.0, "D"=0.0, "F"=0.0, "I Zone"=0.0} ("PIDF"), "P"=0.0, "I"=0.0, "D"=0.0, "F"=0.0, "I Zone"=0.0) -> (w161:T8)
      n54 = Bundle By Name(cluster=T8 {"P"=0.0, "I"=0.0, "D"=0.0, "F"=0.0, "I Zone"=0.0} ("PIDF"), "P"=0.0, "I"=0.0, "D"=0.0, "F"=0.0, "I Zone"=0.0) -> (w229:T8)
      n55 = Bundle By Name(cluster=T12 {"Open Data"={"SRX ID"=0, "Invert Output"=FALSE}, "Current Config Data"={"Enable Current Limit?"=FALSE, "Peak Current (Amps)"=0, "Peak Current Maximum Duration (ms)"=0, "Continuous Current Limit (Amps)"=0}, "Sensor Config"={"Feedback Device"=0, "PhaseSensor"=FALSE}, "Hard Limits"={"Fwd Enable"=FALSE, "Rev Enable"=FALSE, "Fwd NO-NC"=enum."Normally Open", "Rev NO-NC"=enum."Normally Open"}, "Motion Magic Config Data"={"Cruise Velocity"=0, "Acceleration"=0}, "PIDF"={"P"=0.0, "I"=0.0, "D"=0.0, "F"=0.0, "I Zone"=0.0}, "Maximum Integral Accumulator Value"=0.0, "AllowableClosedLoop"=0, "Limits"={"Max"=0, "Min"=0, "Max Enable"=FALSE, "Min Enable"=FALSE}, "Output Config"={"Invert?"=FALSE, "Neutral Mode"=enum."Override to Coast", "Deadband (-1to1)"=0.0, "Ramp Time Off to Full (S)"=0.0, "Peak  (-1to1)"={"Forward"=1.0, "Reverse"=-1.0}, "Nominal  (-1to1)"={"Forward"=0.0, "Reverse"=0.0}}} ("Master"), "Open Data"=w157, "Sensor Config"=w159, "PIDF"=w161, "Maximum Integral Accumulator Value"=0.0, "AllowableClosedLoop"=0, "Limits"=w165, "Output Config"=w167) -> (w153:T12)
      n56 = Bundle By Name(cluster=T12 {"Open Data"={"SRX ID"=0, "Invert Output"=FALSE}, "Current Config Data"={"Enable Current Limit?"=FALSE, "Peak Current (Amps)"=0, "Peak Current Maximum Duration (ms)"=0, "Continuous Current Limit (Amps)"=0}, "Sensor Config"={"Feedback Device"=0, "PhaseSensor"=FALSE}, "Hard Limits"={"Fwd Enable"=FALSE, "Rev Enable"=FALSE, "Fwd NO-NC"=enum."Normally Open", "Rev NO-NC"=enum."Normally Open"}, "Motion Magic Config Data"={"Cruise Velocity"=0, "Acceleration"=0}, "PIDF"={"P"=0.0, "I"=0.0, "D"=0.0, "F"=0.0, "I Zone"=0.0}, "Maximum Integral Accumulator Value"=0.0, "AllowableClosedLoop"=0, "Limits"={"Max"=0, "Min"=0, "Max Enable"=FALSE, "Min Enable"=FALSE}, "Output Config"={"Invert?"=FALSE, "Neutral Mode"=enum."Override to Coast", "Deadband (-1to1)"=0.0, "Ramp Time Off to Full (S)"=0.0, "Peak  (-1to1)"={"Forward"=1.0, "Reverse"=-1.0}, "Nominal  (-1to1)"={"Forward"=0.0, "Reverse"=0.0}}} ("Master"), "Open Data"=w233, "Sensor Config"=w231, "PIDF"=w229, "Maximum Integral Accumulator Value"=0.0, "AllowableClosedLoop"=0, "Limits"=w225, "Output Config"=w223) -> (w237:T12)
      n57 = Bundle By Name(cluster=T12 {"Open Data"={"SRX ID"=0, "Invert Output"=FALSE}, "Current Config Data"={"Enable Current Limit?"=FALSE, "Peak Current (Amps)"=0, "Peak Current Maximum Duration (ms)"=0, "Continuous Current Limit (Amps)"=0}, "Sensor Config"={"Feedback Device"=0, "PhaseSensor"=FALSE}, "Hard Limits"={"Fwd Enable"=FALSE, "Rev Enable"=FALSE, "Fwd NO-NC"=enum."Normally Open", "Rev NO-NC"=enum."Normally Open"}, "Motion Magic Config Data"={"Cruise Velocity"=0, "Acceleration"=0}, "PIDF"={"P"=0.0, "I"=0.0, "D"=0.0, "F"=0.0, "I Zone"=0.0}, "Maximum Integral Accumulator Value"=0.0, "AllowableClosedLoop"=0, "Limits"={"Max"=0, "Min"=0, "Max Enable"=FALSE, "Min Enable"=FALSE}, "Output Config"={"Invert?"=FALSE, "Neutral Mode"=enum."Override to Coast", "Deadband (-1to1)"=0.0, "Ramp Time Off to Full (S)"=0.0, "Peak  (-1to1)"={"Forward"=1.0, "Reverse"=-1.0}, "Nominal  (-1to1)"={"Forward"=0.0, "Reverse"=0.0}}} ("Master"), "Open Data.SRX ID"=u8 5, "Open Data.Invert Output"=FALSE) -> (w152:T12)
      n58 = Bundle By Name(cluster=T12 {"Open Data"={"SRX ID"=0, "Invert Output"=FALSE}, "Current Config Data"={"Enable Current Limit?"=FALSE, "Peak Current (Amps)"=0, "Peak Current Maximum Duration (ms)"=0, "Continuous Current Limit (Amps)"=0}, "Sensor Config"={"Feedback Device"=0, "PhaseSensor"=FALSE}, "Hard Limits"={"Fwd Enable"=FALSE, "Rev Enable"=FALSE, "Fwd NO-NC"=enum."Normally Open", "Rev NO-NC"=enum."Normally Open"}, "Motion Magic Config Data"={"Cruise Velocity"=0, "Acceleration"=0}, "PIDF"={"P"=0.0, "I"=0.0, "D"=0.0, "F"=0.0, "I Zone"=0.0}, "Maximum Integral Accumulator Value"=0.0, "AllowableClosedLoop"=0, "Limits"={"Max"=0, "Min"=0, "Max Enable"=FALSE, "Min Enable"=FALSE}, "Output Config"={"Invert?"=FALSE, "Neutral Mode"=enum."Override to Coast", "Deadband (-1to1)"=0.0, "Ramp Time Off to Full (S)"=0.0, "Peak  (-1to1)"={"Forward"=1.0, "Reverse"=-1.0}, "Nominal  (-1to1)"={"Forward"=0.0, "Reverse"=0.0}}} ("Master"), "Open Data.SRX ID"=u8 2, "Open Data.Invert Output"=FALSE) -> (w236:T12)
      n59 = Bundle By Name(cluster=T16 {"Left Master"={"Open Data"={"SRX ID"=0, "Invert Output"=FALSE}, "Current Config Data"={"Enable Current Limit?"=FALSE, "Peak Current (Amps)"=0, "Peak Current Maximum Duration (ms)"=0, "Continuous Current Limit (Amps)"=0}, "Sensor Config"={"Feedback Device"=1, "PhaseSensor"=FALSE}, "Hard Limits"={"Fwd Enable"=FALSE, "Rev Enable"=FALSE, "Fwd NO-NC"=enum."Normally Open", "Rev NO-NC"=enum."Normally Open"}, "Motion Magic Config Data"={"Cruise Velocity"=0, "Acceleration"=0}, "PIDF"={"P"=0.0, "I"=0.0, "D"=0.0, "F"=0.0, "I Zone"=0.0}, "Maximum Integral Accumulator Value"=0.0, "AllowableClosedLoop"=0, "Limits"={"Max"=0, "Min"=0, "Max Enable"=FALSE, "Min Enable"=FALSE}, "Output Config"={"Invert?"=FALSE, "Neutral Mode"=enum."EEPROMSetting", "Deadband (-1to1)"=0.0, "Ramp Time Off to Full (S)"=0.0, "Peak  (-1to1)"={"Forward"=1.0, "Reverse"=-1.0}, "Nominal  (-1to1)"={"Forward"=0.0, "Reverse"=0.0}}}, "Right Master"={"Open Data"={"SRX ID"=0, "Invert Output"=FALSE}, "Current Config Data"={"Enable Current Limit?"=FALSE, "Peak Current (Amps)"=0, "Peak Current Maximum Duration (ms)"=0, "Continuous Current Limit (Amps)"=0}, "Sensor Config"={"Feedback Device"=1, "PhaseSensor"=FALSE}, "Hard Limits"={"Fwd Enable"=FALSE, "Rev Enable"=FALSE, "Fwd NO-NC"=enum."Normally Open", "Rev NO-NC"=enum."Normally Open"}, "Motion Magic Config Data"={"Cruise Velocity"=0, "Acceleration"=0}, "PIDF"={"P"=0.0, "I"=0.0, "D"=0.0, "F"=0.0, "I Zone"=0.0}, "Maximum Integral Accumulator Value"=0.0, "AllowableClosedLoop"=0, "Limits"={"Max"=0, "Min"=0, "Max Enable"=FALSE, "Min Enable"=FALSE}, "Output Config"={"Invert?"=FALSE, "Neutral Mode"=enum."EEPROMSetting", "Deadband (-1to1)"=0.0, "Ramp Time Off to Full (S)"=0.0, "Peak  (-1to1)"={"Forward"=1.0, "Reverse"=-1.0}, "Nominal  (-1to1)"={"Forward"=0.0, "Reverse"=0.0}}}, "Left Slave"={"Open Data"={"SRX ID"=0, "Invert Output"=FALSE}, "Current Config Data"={"Enable Current Limit?"=FALSE, "Peak Current (Amps)"=0, "Peak Current Maximum Duration (ms)"=0, "Continuous Current Limit (Amps)"=0}, "Sensor Config"={"Feedback Device"=1, "PhaseSensor"=FALSE}, "Hard Limits"={"Fwd Enable"=FALSE, "Rev Enable"=FALSE, "Fwd NO-NC"=enum."Normally Open", "Rev NO-NC"=enum."Normally Open"}, "Motion Magic Config Data"={"Cruise Velocity"=0, "Acceleration"=0}, "PIDF"={"P"=0.0, "I"=0.0, "D"=0.0, "F"=0.0, "I Zone"=0.0}, "Maximum Integral Accumulator Value"=0.0, "AllowableClosedLoop"=0, "Limits"={"Max"=0, "Min"=0, "Max Enable"=FALSE, "Min Enable"=FALSE}, "Output Config"={"Invert?"=FALSE, "Neutral Mode"=enum."EEPROMSetting", "Deadband (-1to1)"=0.0, "Ramp Time Off to Full (S)"=0.0, "Peak  (-1to1)"={"Forward"=1.0, "Reverse"=-1.0}, "Nominal  (-1to1)"={"Forward"=0.0, "Reverse"=0.0}}}, "Right Slave"={"Open Data"={"SRX ID"=0, "Invert Output"=FALSE}, "Current Config Data"={"Enable Current Limit?"=FALSE, "Peak Current (Amps)"=0, "Peak Current Maximum Duration (ms)"=0, "Continuous Current Limit (Amps)"=0}, "Sensor Config"={"Feedback Device"=1, "PhaseSensor"=FALSE}, "Hard Limits"={"Fwd Enable"=FALSE, "Rev Enable"=FALSE, "Fwd NO-NC"=enum."Normally Open", "Rev NO-NC"=enum."Normally Open"}, "Motion Magic Config Data"={"Cruise Velocity"=0, "Acceleration"=0}, "PIDF"={"P"=0.0, "I"=0.0, "D"=0.0, "F"=0.0, "I Zone"=0.0}, "Maximum Integral Accumulator Value"=0.0, "AllowableClosedLoop"=0, "Limits"={"Max"=0, "Min"=0, "Max Enable"=FALSE, "Min Enable"=FALSE}, "Output Config"={"Invert?"=FALSE, "Neutral Mode"=enum."EEPROMSetting", "Deadband (-1to1)"=0.0, "Ramp Time Off to Full (S)"=0.0, "Peak  (-1to1)"={"Forward"=1.0, "Reverse"=-1.0}, "Nominal  (-1to1)"={"Forward"=0.0, "Reverse"=0.0}}}} ("Drive Setup"), "Left Master"=w237, "Left Slave"=w236, "Right Master"=w153, "Right Slave"=w152) -> (w151:T16)
      n60 = global write "Global_Device_IDs.vi" "Drive Setup"(w151) -> ()
    }
    frame Disabled {
    }
  }
  n61 = disable-structure shown="Enabled" {
    frame Enabled {
      n62 = Bundle By Name(cluster=T19 {"Left Motor Setup"={"Motor ID"=0, "Invert Motor"=FALSE}, "Right Motor Setup"={"Motor ID"=0, "Invert Motor"=FALSE}, "Left Motor PDP"=0, "Right Motor PDP"=0, "Solonoid Setup"={"Pneumatics Control Module (0)"=0, "Forward Solenoid Channel"=enum."Solenoid 0", "Reverse Solenoid Channel"=enum."Solenoid 0"}, "Limit Switch DIO"=enum."DIO 0"} ("Claw Setup"), "Left Motor Setup.Motor ID"=u8 11, "Left Motor Setup.Invert Motor"=TRUE, "Left Motor PDP"=0, "Right Motor Setup.Motor ID"=u8 12, "Right Motor Setup.Invert Motor"=FALSE, "Right Motor PDP"=0, "Solonoid Setup.Pneumatics Control Module (0)"=u8 0, "Solonoid Setup.Forward Solenoid Channel"=WPI_SolenoidChannel."Solenoid 2", "Solonoid Setup.Reverse Solenoid Channel"=WPI_SolenoidChannel."Solenoid 3", "Limit Switch DIO"=FPGA_DIOChannel."DIO 0") -> (w249:T19)
      n63 = global write "Global_Device_IDs.vi" "Claw Setup"(w249) -> ()
    }
    frame Disabled {
    }
  }
  "error out" <- "error in"
